vi "HotLotRun.vi"() -> ()   [LabVIEW 2012]
uses:
  <vilib>/Utility/NIReport.llb/NI_report.lvclass
  Global1.vi
  <vilib>/Utility/NIReport.llb/Excel/NI_Excel.lvclass
panel:
  out "Array":string[][](array[string])
  out "error out 2":errorcluster
  out "error out":errorcluster
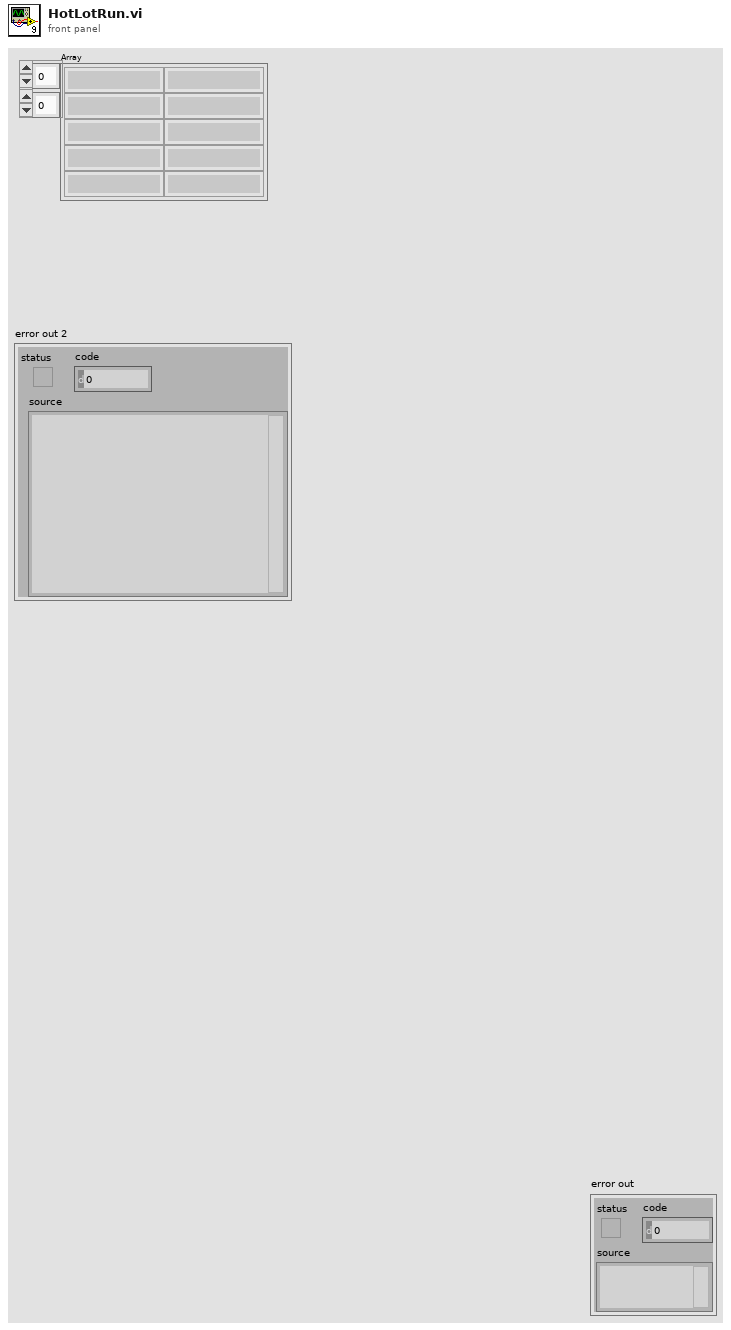
[diagram p1: front panel]
types:
  T1 = enum16{"Standard Report", "HTML", "Word", "Excel"}
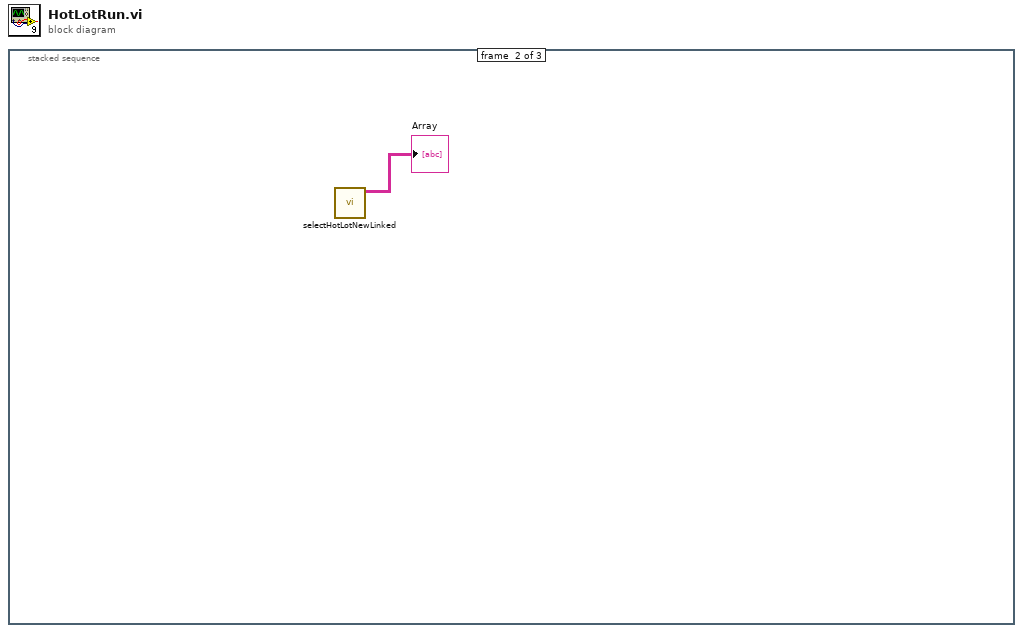
[diagram p0: block diagram]
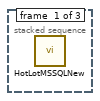
[diagram p2: hidden frame]
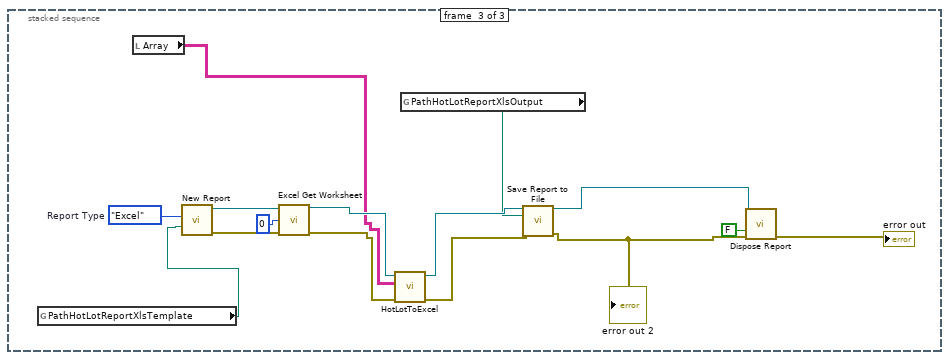
[diagram p3: hidden frame]
diagram:
  n1 = stacked-sequence {
    frame #0 {
      n2 = call "HotLotMSSQLNew.vi"() -> ()  [unwired: 12 in]
    }
    frame #1 {
      n3 = call "selectHotLotNewLinked.vi"() -> ("Array"=→"Array":string[][])  [unwired: 10 in, 1 out]
    }
    frame #2 {
      w16 = T1."Excel"  # Report Type
      n4 = global read "Global1.vi" "PathHotLotReportXlsTemplate"() -> (w12:path)
      n5 = local read "Array"() -> (w3:string[][])
      n6 = call <vilib>:"New Report.vi"("report type"=w16, "template (empty)"=w12) -> ("report out"=w15:refnum<class "NI_report.lvclass">, "error out"=w14:errorcluster)  [unwired: 12 in]
      n7 = call <vilib>:"Excel Get Worksheet.vi"("report in"=w15, "worksheet index (0)"=0, "error in (no error)"=w14) -> ("report out"=w7:refnum<class "NI_report.lvclass">, "error out"=w6:errorcluster)  [unwired: 11 in]
      n8 = call "HotLotToExcel.vi"("error in (no error)"=w6, "Input"=w3, "report in"=w7) -> ("error out"=w4:errorcluster, "report out"=w5:refnum<class "NI_report.lvclass">)  [unwired: 7 in]
      n9 = global read "Global1.vi" "PathHotLotReportXlsOutput"() -> (w2:path)
      n10 = call-dynamic "Save Report to File.vi"("report in"=w5, "report file path"=w2, "error in (no error)"=w4) -> ("report out"=w11:refnum<class "NI_report.lvclass">, "error out"=w10:errorcluster)  [unwired: 11 in]
      "error out 2" <- w10
      n11 = call-dynamic "Dispose Report.vi"("report in"=w11, "save changes? (F)"=FALSE, "error in (no error)"=w10) -> ("error out"=→"error out":errorcluster)  [unwired: 12 in]
    }
  }
